vi "Read Path.vi"(7 "key":string, 8 "error in (no error)":errorcluster, 9 "default value":path, 11 "Configuration File In":refnum<class "Configuration File.lvclass">) -> (0 "error out":errorcluster, 1 "value":path, 3 "Configuration File Out":refnum<class "Configuration File.lvclass">)   [LabVIEW 2020, in "Configuration File.lvclass"]
doc: "High-level function for reading configuration file data from process class. If the specified key is not present, it is added with the configured default value."
uses:
  Configuration File.lvclass
  <vilib>/Utility/config.llb/NI_LVConfig.lvlib
  <vilib>/Utility/config.llb/Read Key (Path).vi
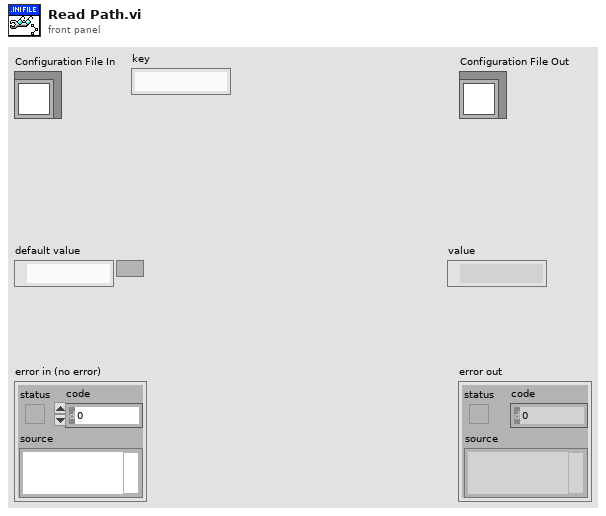
[diagram p1: front panel]
types:
  T1 = typedef "NI_LVConfig.lvlib/Config Data RefNum.ctl" = refnum<k1>
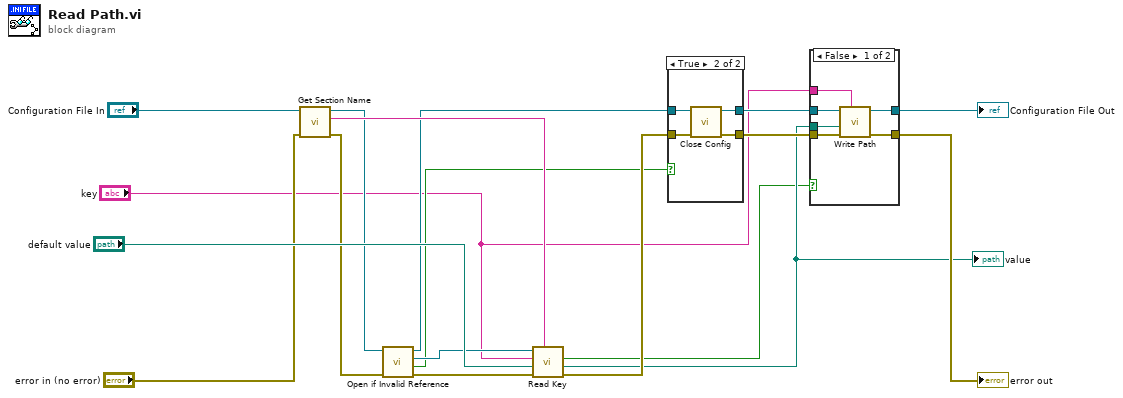
[diagram p0: block diagram]
diagram:
  n1 = call "Get Section Name.vi"("error in (no error)"="error in (no error)", "Configuration File In"="Configuration File In") -> ("error out"=w13:errorcluster, "Section Name"=w17:string, "Configuration File Out"=w10:refnum<class "Configuration File.lvclass">)  [unwired: 7 in]
  n2 = call "Open if Invalid Reference.vi"("error in (no error)"=w13, "Configuration File In"=w10) -> ("error out"=w12:errorcluster, "File opened?"=w2:bool, "refnum out"=w14:T1, "Configuration File Out"=w11:refnum<class "Configuration File.lvclass">)  [unwired: 6 in]
  n3 = call-poly <vilib>:"Read Key.vi"("section"=w17, "error in (no error)"=w12, "default value"="default value", "key"="key", "refnum"=w14) -> ("error out"=w6:errorcluster, "value"=w4:path, "found?"=w3:bool)  [unwired: 3 in, 1 out]
  "value" <- w4
  n4 = case shown="True" w2 {
    tunnel: w11 -> [w20 w24]
    tunnel: [w20 w23] -> w9
    tunnel: [w19 w22] -> w7
    tunnel: w6 -> [w19 w21]
    frame False {
    }
    frame True {
      n5 = call-dynamic "Close Config.vi"("error in (no error)"=w21, "Configuration File File In"=w24) -> ("error out"=w22:errorcluster, "Configuration File File Out"=w23:refnum<class "Configuration File.lvclass">)  [unwired: 8 in]
    }
  }
  n6 = case shown="False" w3 {
    tunnel: w9 -> [w30 w32]
    tunnel: [w29 w32] -> w8
    tunnel: w7 -> [w28 w31]
    tunnel: [w27 w31] -> w5
    tunnel: w4 -> [w26 _]
    tunnel: "key" -> [w25 _]
    frame False {
      n7 = call-dynamic "Write Path.vi"("key"=w25, "error in (no error)"=w28, "Value"=w26, "Configuration File In"=w30) -> ("error out"=w27:errorcluster, "Configuration File Out"=w29:refnum<class "Configuration File.lvclass">)  [unwired: 6 in]
    }
    frame True {
    }
  }
  "error out" <- w5
  "Configuration File Out" <- w8
